vi "接收硬件返回的数据.vi"(8 "error in (no error)":errorcluster caption="错误输入（无错误）", 11 "客户端 输入":refnum<class "客户端.lvclass">) -> (0 "error out":errorcluster caption="错误输出", 2 "硬件返回的数据":string, 3 "客户端 输出":refnum<class "客户端.lvclass">)   [LabVIEW 2015, in "客户端.lvlib" / "客户端.lvclass"]
uses:
  <vilib>/Instr/_visa.llb/VISA Configure Serial Port (Instr).vi
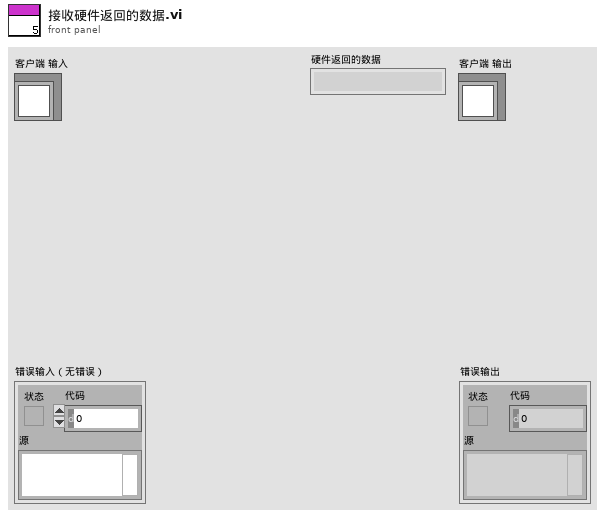
[diagram p1: front panel]
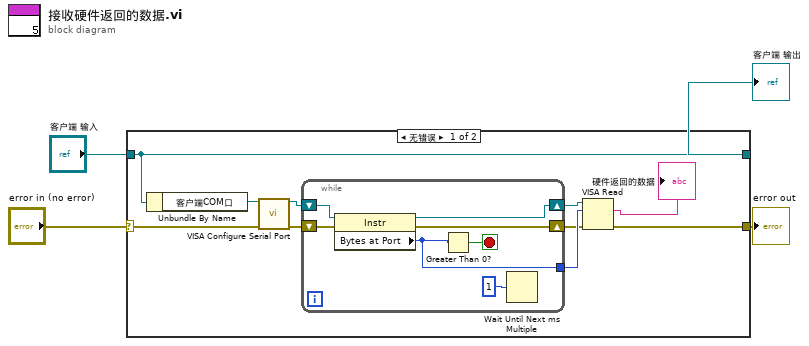
[diagram p0: block diagram]
diagram:
  n1 = case shown="无错误" "error in (no error)" {
    selector: "error in (no error)" -> [w12 w23]
    tunnel: [w5 w23] -> w3
    tunnel: [w14 w22] -> w1
    tunnel: "客户端 输入" -> [w14 w22]
    frame No Error {
      n2 = Unbundle By Name(w14) -> ("客户端COM口"=w13:refnum<visa-resource-name>)
      n3 = call-poly "VISA Configure Serial Port"("VISA resource name"=w13, "error in (no error)"=w12) -> ("VISA resource name out"=w11:refnum<visa-resource-name>, "error out"=w10:errorcluster)  [unwired: 12 in]
      n4 = while {
        tunnel: [w15] -> w9
        shift-right: [w19] -> w8
        shift-left: w11 -> [w21]
        shift-right: [w18] -> w7
        shift-left: w10 -> [w20]
        stop <- w16 stop-if-true
        n5 = property class="Instr"(reference=w21, error in=w20) -> (reference out=w19:refnum<visa-resource-name>, error out=w18:errorcluster, "Bytes at Port"=w15:u32)
        n6 = Greater Than 0?(x=w15) -> (x > 0?=w16:bool)
        n7 = Wait Until Next ms Multiple(millisecond multiple=u32 1 ("毫秒倍数")) -> ()  [unwired: 1 out]
      }
      n8 = VISA Read(VISA resource name=w8, byte count=w9, error in (no error)=w7) -> (read buffer=→"硬件返回的数据":string, error out=w5:errorcluster)  [unwired: 2 out]
    }
    frame Error {
    }
  }
  "error out" <- w3
  "客户端 输出" <- w1
